vi "VIBRATION_SENSOR.vi"() -> (0 "Numeric":dbl, 1 "Waveform Chart":dbl(graph))   [LabVIEW 2014]
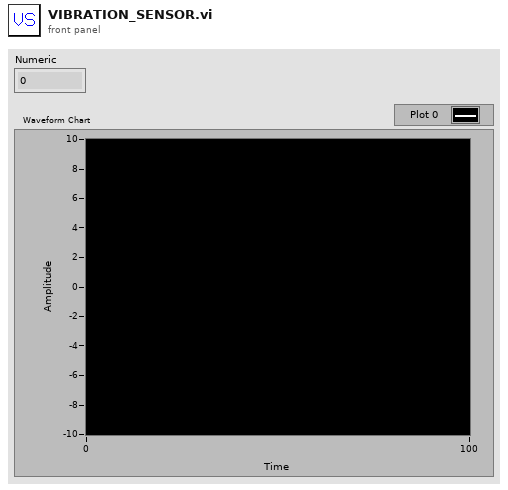
[diagram p1: front panel]
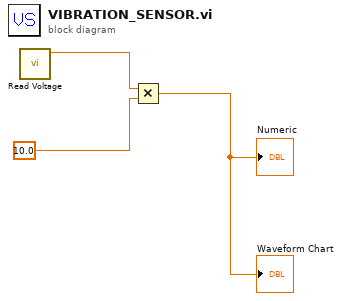
[diagram p0: block diagram]
diagram:
  n1 = call "Read Voltage.vi"() -> ("voltage"=w2:dbl)  [unwired: 6 in, 1 out]
  n2 = Multiply(x=w2, y=10.0) -> (x*y=→"Numeric" →"Waveform Chart":dbl)
